vi "myRIOXGenerateVIName.vi"(8 "error in (no error)":errorcluster, 10 "Original VI Name":string, 11 "VI Refnum In":refnum<vi>) -> (0 "error out":errorcluster, 2 "Proposed VI Name":string, 3 "VI Refnum Out":refnum<vi>)   [LabVIEW 2021]
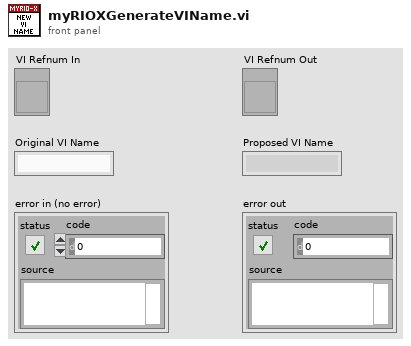
[diagram p1: front panel]
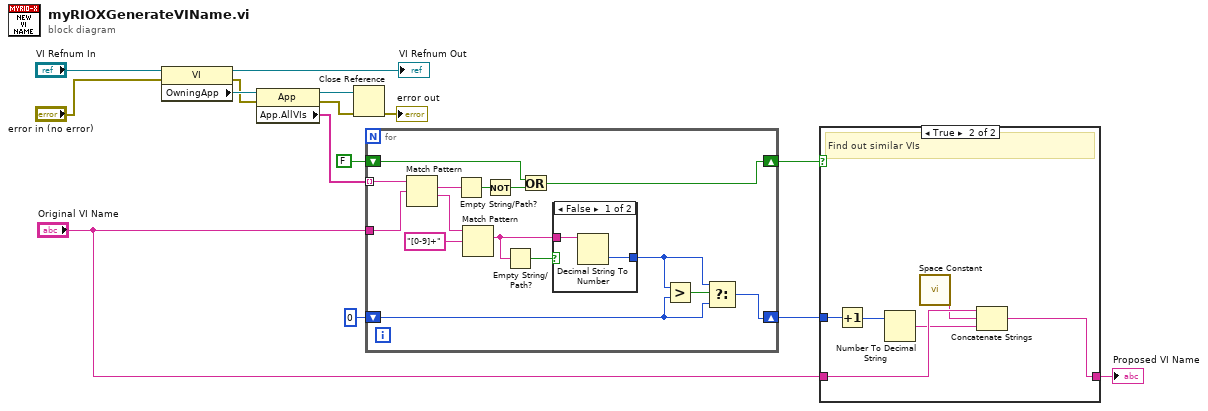
[diagram p0: block diagram]
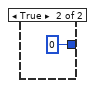
[diagram p3: hidden frame]
diagram:
  n1 = property class="VI"(reference="VI Refnum In", error in="error in (no error)") -> (reference out=→"VI Refnum Out":refnum<vi>, error out=w12:errorcluster, "OwningApp"=w13:refnum<vi>)
  n2 = property class="App"(reference=w13, error in=w12) -> (reference out=w9:refnum<vi>, error out=w8:errorcluster, "App.AllVIs"=w10:string[])
  n3 = Close Reference(reference=w9, error in (no error)=w8) -> (error out=→"error out":errorcluster)
  n4 = for {
    tunnel: w10 -> [w30] mode=indexing
    tunnel: "Original VI Name" -> [w29]
    shift-right: [w24] -> w4
    shift-left: FALSE -> [w25]
    shift-right: [w16] -> w3
    shift-left: u32 0 -> [w18]
    n5 = Match Pattern(string=w30, regular expression=w29) -> (match substring=w28:string, after substring=w23:string)  [unwired: 1 in, 2 out]
    n6 = Empty String/Path?(string/path=w28) -> (empty?=w27:bool)
    n7 = Match Pattern(string=w23, regular expression="[0-9]+") -> (match substring=w20:string)  [unwired: 1 in, 3 out]
    n8 = Not(x=w27) -> (.not. x?=w26:bool)
    n9 = Empty String/Path?(string/path=w20) -> (empty?=w21:bool)
    n10 = Or(x=w25, y=w26) -> (x .or. y?=w24:bool)
    n11 = case shown="False" w21 {
      tunnel: w20 -> [w32 _]
      tunnel: [w31 u32 0] -> w17
      frame False {
        n12 = Decimal String To Number(string=w32) -> (number=w31:i32)  [unwired: 2 in, 1 out]
      }
      frame True {
      }
    }
    n13 = Greater?(x=w17, y=w18) -> (0:w19:bool)
    n14 = Select(t=w17, s=w19, f=w18) -> (s? t:f=w16:u32)
  }
  n15 = case shown="True" w4 {
    tunnel: w3 -> [_ w40]
    tunnel: "Original VI Name" -> [w34 w38]
    tunnel: [w34 w35] -> w1
    frame False {
      # "Do not find out any existing VI with similar name"
    }
    frame True {
      # "Find out similar VIs"
      n16 = Increment(x=w40) -> (x+1=w39:u32)
      n17 = Number To Decimal String(number=w39) -> (decimal integer string=w37:string)  [unwired: 1 in]
      n18 = call <vilib>:"Space Constant.vi"() -> ("String"=w36:string)
      n19 = Concatenate Strings(w38, w36, w37) -> (w35:string)
    }
  }
  "Proposed VI Name" <- w1
